vi "Kitchen Timer.vi"() -> ()   [LabVIEW 2020]
panel:
  in  "Timer set(s)":i32(knob) scale=0.0..10.0
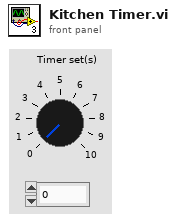
[diagram p1: front panel]
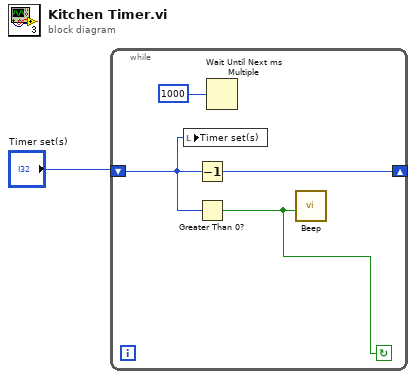
[diagram p0: block diagram]
diagram:
  n1 = while {
    shift-right: [w4] -> _
    shift-left: "Timer set(s)" -> [w3]
    stop <- w2 continue-if-true
    n2 = local write "Timer set(s)"(w3) -> ()
    n3 = Decrement(x=w3) -> (x-1=w4:i32)
    n4 = Greater Than 0?(x=w3) -> (x > 0?=w2:bool)
    n5 = Wait Until Next ms Multiple(millisecond multiple=u32 1000 ("millisecond timer value")) -> ()  [unwired: 1 out]
    n6 = call <vilib>:"Beep.vi"("use system alert? (T)"=w2) -> ()  [unwired: 11 in]
  }
